vi "Vision Steering.vi"() -> ()   [LabVIEW 2015]
uses:
  <vilib>/Rock Robotics/Network Tables/NT Read Number.vi
panel:
  in  "stop":bool
  in  "array":T1(array[cluster])
  out "Meter":dbl(knob) scale=-32.0..32.0
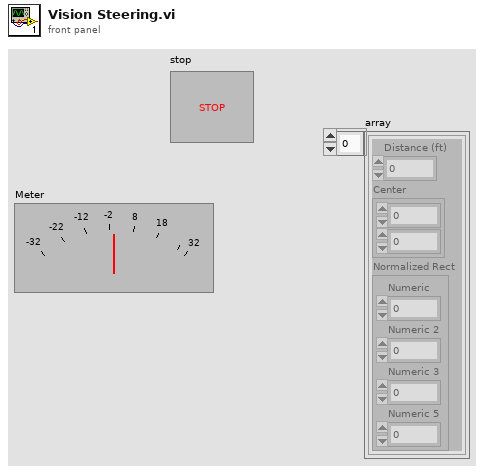
[diagram p1: front panel]
types:
  T1 = cluster{"Distance (ft)":dbl, "Center":cluster{dbl, dbl}, "Normalized Rect":cluster{"Numeric":dbl, "Numeric 2":dbl, "Numeric 3":dbl, "Numeric 5":dbl}}[]
  T2 = cluster{"Distance (ft)":dbl, "Center":cluster{dbl, dbl}, "Normalized Rect":cluster{"Numeric":dbl, "Numeric 2":dbl, "Numeric 3":dbl, "Numeric 5":dbl}}
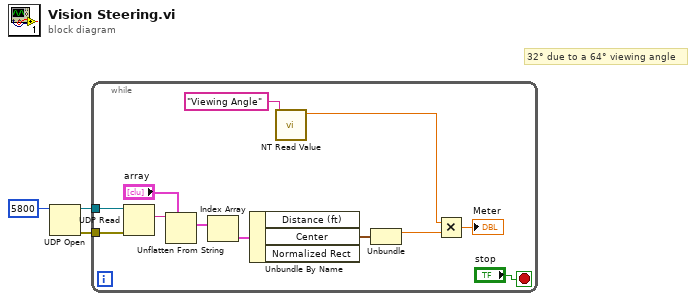
[diagram p0: block diagram]
diagram:
  # "32° due to a 64° viewing angle"
  n1 = UDP Open(11:u16 5800 ("port")) -> (port=w2:refnum<k16>, 0:w1:errorcluster)  [unwired: 4 in, 1 out]
  n2 = while {
    tunnel: w2 -> [w14]
    tunnel: w1 -> [w7]
    stop <- "stop" stop-if-true
    n3 = UDP Read(connection ID=w14, 8:w7) -> (data out=w13:string)  [unwired: 2 in, 4 out]
    n4 = Unflatten From String(type="array", binary string=w13) -> (value=w11:T1)  [unwired: 3 in, 2 out]
    n5 = Index Array(array=w11) -> (element=w10:T2)  [unwired: 1 in]
    n6 = Unbundle By Name(w10) -> ("Center"=w9:cluster{dbl, dbl})  [unwired: 2 out]
    n7 = call-poly <vilib>:"NT Read Value.vi"("Name"="Viewing Angle") -> ("Numeric"=w5:dbl)  [unwired: 9 in, 1 out]
    n8 = Unbundle(w9) -> (w8:dbl)  [unwired: 1 out]
    n9 = Multiply(x=w5, y=w8) -> (x*y=→"Meter":dbl)
  }
